vi "test-twist2d.vi"() -> (3 "All PASSED":bool)   [LabVIEW 2019]
uses:
  <vilib>/Rock Robotics/WPI/ThirdParty/JAS_Junk/TrajLib/Rotation_CreateAngle.vi
  <vilib>/Rock Robotics/WPI/ThirdParty/JAS_Junk/TrajLib/Translation_Create.vi
  <vilib>/Rock Robotics/WPI/ThirdParty/JAS_Junk/TrajLib/Trajectory_Library.lvlib
panel:
  out "T3 - Theta - 0":dbl
  out "T3 - X - 0":dbl
  out "T3 - Y - 0":dbl
  out "T2 - Equals - False":bool
  out "T1 - Equals - True":bool
  out "T0 -- Deg -- 0":dbl
  out "T0 -- y -- 0":dbl
  out "T0 -- X -- 0":dbl
  # "Twist2D Test"
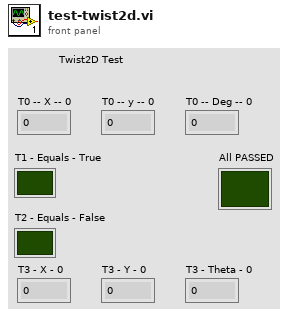
[diagram p1: front panel]
types:
  T1 = typedef "Trajectory_Library.lvlib/POSE2D.ctl" = cluster{"TRANSLATION":T2, "ROTATION":T3}
  T2 = typedef "Trajectory_Library.lvlib/TRANSLATION2D.ctl" = cluster{"X":dbl, "Y":dbl}
  T3 = typedef "Trajectory_Library.lvlib/ROTATION2D.ctl" = cluster{"VALUE":dbl, "COS":dbl, "SIN":dbl}
  T4 = typedef "Trajectory_Library.lvlib/TWIST2D.ctl" = cluster{"dX":dbl, "dY":dbl, "dTHETA":dbl}
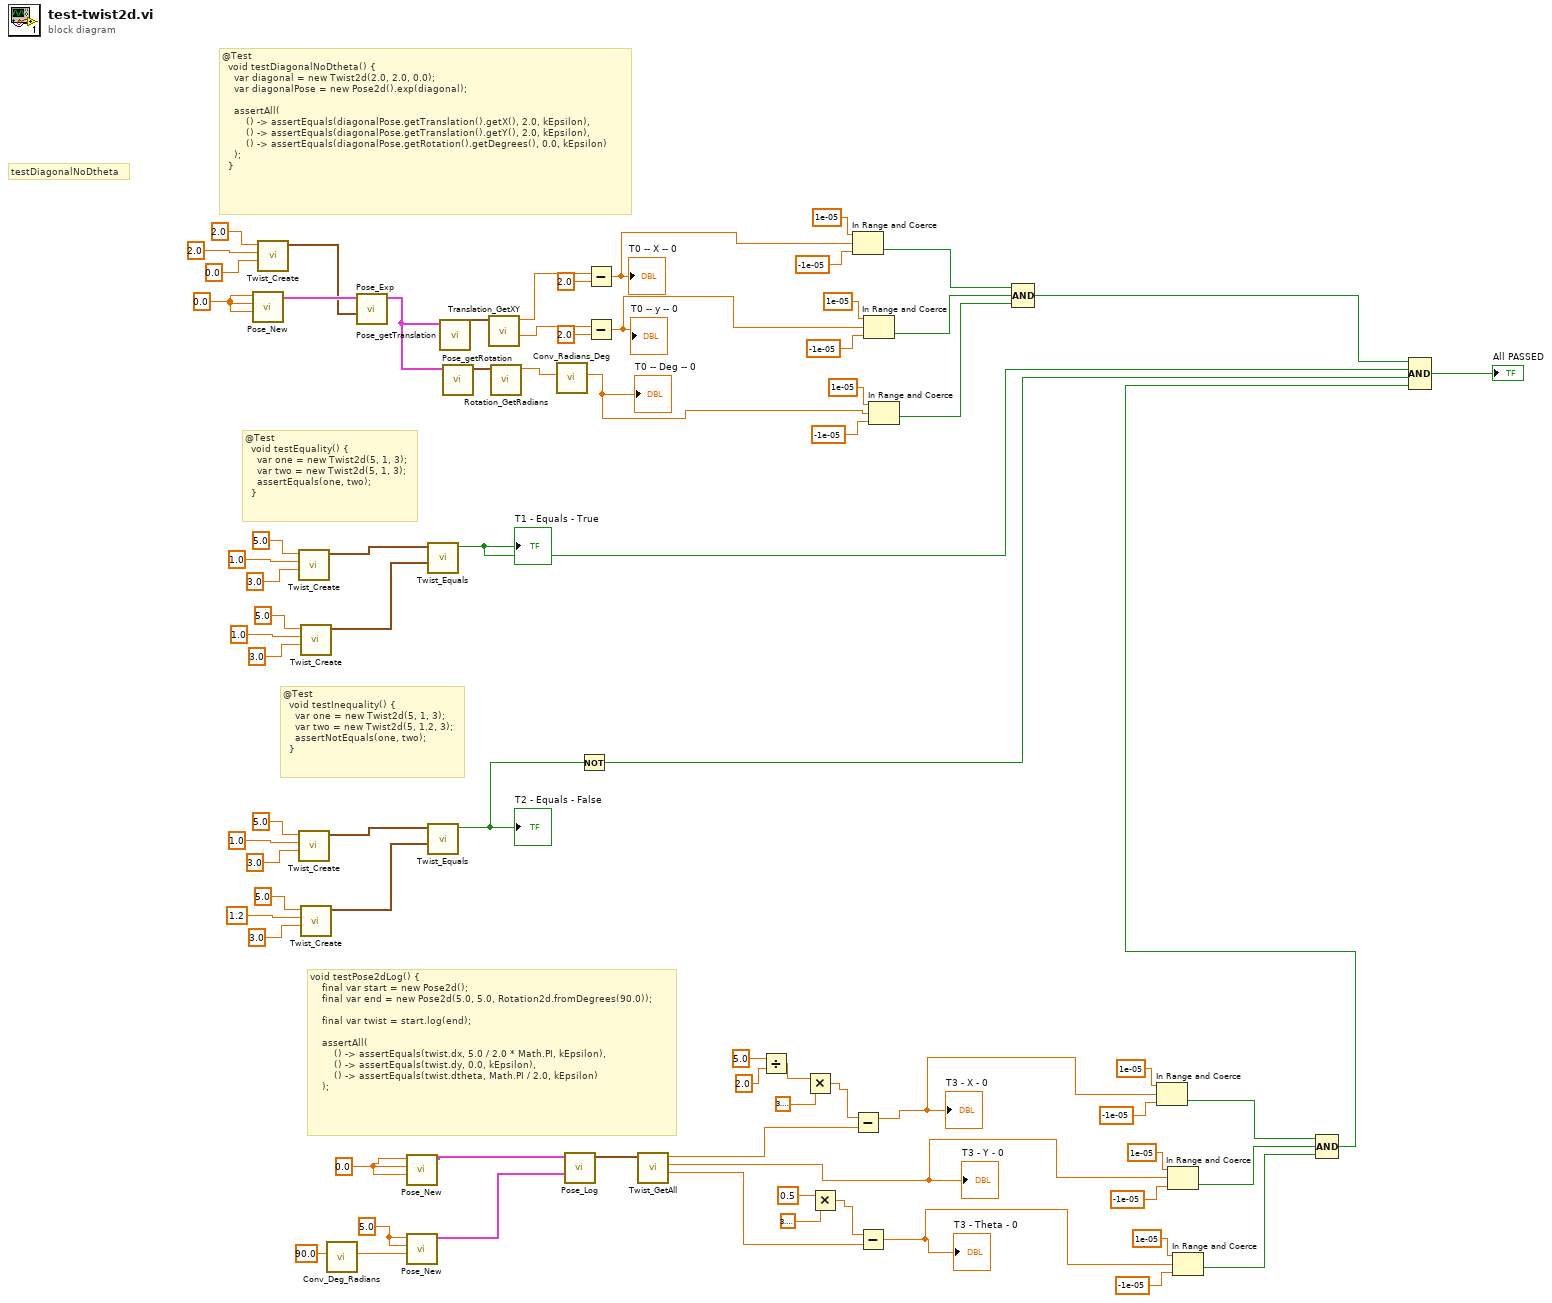
[diagram p0: block diagram]
diagram:
  w46 = 5.0 ("X")
  w31 = 0.0 ("X")
  w74 = 0.0 ("X")
  # "void testPose2dLog() {\n    final var start = new Pose2d();\n    final var end = new Pose2d(5.0, 5.0, Rotation2d.fromDegrees(90.0));\n\n    final var twist = start.log(end);\n\n    assertAll(\n        () -> assertEquals(twist.dx, 5.0 / 2.0 * Math.PI, kEpsilon),\n        () -> assertEquals(twist.dy, 0.0, kEpsilon),\n        () -> assertEquals(twist.dtheta, Math.PI / 2.0, kEpsilon)\n    );"
  # "@Test\n  void testInequality() {\n    var one = new Twist2d(5, 1, 3);\n    var two = new Twist2d(5, 1.2, 3);\n    assertNotEquals(one, two);\n  }"
  # "@Test\n  void testEquality() {\n    var one = new Twist2d(5, 1, 3);\n    var two = new Twist2d(5, 1, 3);\n    assertEquals(one, two);\n  }"
  # "@Test\n  void testDiagonalNoDtheta() {\n    var diagonal = new Twist2d(2.0, 2.0, 0.0);\n    var diagonalPose = new Pose2d().exp(diagonal);\n\n    assertAll(\n        () -> assertEquals(diagonalPose.getTranslation().getX(), 2.0, kEpsilon),\n        () -> assertEquals(diagonalPose.getTranslation().getY(), 2.0, kEpsilon),\n        () -> assertEquals(diagonalPose.getRotation().getDegrees(), 0.0, kEpsilon)\n    );\n  }"
  # "testDiagonalNoDtheta"
  n1 = call <vilib>:"Pose_New.vi"("Heading"=w74, "Y"=w74, "X"=w74) -> ("out POSe"=w73:T1)  [unwired: 8 in]
  n2 = call <vilib>:"Twist_Create.vi"("dTHETA"=0.0, "dY"=2.0, "dX"=2.0) -> ("TWIST"=w72:T4)  [unwired: 8 in]
  n3 = call <vilib>:"Twist_Create.vi"("dTHETA"=3.0, "dY"=1.0, "dX"=5.0) -> ("TWIST"=w57:T4)  [unwired: 8 in]
  n4 = call <vilib>:"Twist_Create.vi"("dTHETA"=3.0, "dY"=1.0, "dX"=5.0) -> ("TWIST"=w49:T4)  [unwired: 8 in]
  n5 = call <vilib>:"Twist_Create.vi"("dTHETA"=3.0, "dY"=1.0, "dX"=5.0) -> ("TWIST"=w56:T4)  [unwired: 8 in]
  n6 = call <vilib>:"Twist_Create.vi"("dTHETA"=3.0, "dY"=1.2, "dX"=5.0) -> ("TWIST"=w48:T4)  [unwired: 8 in]
  n7 = call <vilib>:"Conv_Deg_Radians.vi"("Degress"=90.0) -> ("Radians"=w45:dbl)  [unwired: 10 in]
  n8 = call <vilib>:"Pose_Exp.vi"("TWIST"=w72, "POSE"=w73) -> ("UpdatedPose"=w71:T1)  [unwired: 9 in]
  n9 = call <vilib>:"Pose_New.vi"("Heading"=w31, "Y"=w31, "X"=w31) -> ("out POSe"=w44:T1)  [unwired: 8 in]
  n10 = call <vilib>:"Pose_New.vi"("Heading"=w45, "Y"=w46, "X"=w46) -> ("out POSe"=w43:T1)  [unwired: 8 in]
  n11 = call <vilib>:"Twist_Equals.vi"("other TWIST"=w56, "this TWIST"=w57) -> ("Equals"=w3:bool)  [unwired: 9 in]
  "T1 - Equals - True" <- w3
  n12 = call <vilib>:"Twist_Equals.vi"("other TWIST"=w48, "this TWIST"=w49) -> ("Equals"=w4:bool)  [unwired: 9 in]
  "T2 - Equals - False" <- w4
  n13 = call <vilib>:"Pose_getTranslation.vi"("in POSE"=w71) -> ("outTRANSLATION"=w70:T2)  [unwired: 10 in]
  n14 = call <vilib>:"Pose_getRotation.vi"("in POSE"=w71) -> ("out ROTATION"=w69:T3)  [unwired: 10 in]
  n15 = call <vilib>:"Translation_GetXY.vi"("In Translation"=w70) -> ("Y"=w65:dbl, "X"=w68:dbl)  [unwired: 9 in]
  n16 = call <vilib>:"Rotation_GetRadians.vi"("in ROTATION"=w69) -> ("AngleRadians"=w64:dbl)  [unwired: 10 in]
  n17 = call <vilib>:"Conv_Radians_Deg.vi"("Radians"=w64) -> ("Degrees"=w18:dbl)  [unwired: 10 in]
  "T0 -- Deg -- 0" <- w18
  n18 = call <vilib>:"Pose_Log.vi"("end POSE"=w43, "in POSE"=w44) -> ("out TWIST"=w42:T4)  [unwired: 9 in]
  n19 = Not(x=w4) -> (.not. x?=w2:bool)
  n20 = Subtract(x=w68, y=2.0) -> (x-y=w17:dbl)
  "T0 -- X -- 0" <- w17
  n21 = Subtract(x=w65, y=2.0) -> (x-y=w19:dbl)
  "T0 -- y -- 0" <- w19
  n22 = call <vilib>:"Twist_GetAll.vi"("TWIST"=w42) -> ("dTHETA"=w32:dbl, "dY"=w6:dbl, "dX"=w36:dbl)  [unwired: 8 in]
  "T3 - Y - 0" <- w6
  n23 = Divide(x=5.0, y=2.0) -> (x/y=w38:dbl)
  n24 = Multiply(x=w38, y=3.141592653589793) -> (x*y=w37:dbl)
  n25 = Multiply(x=0.5, y=3.141592653589793) -> (x*y=w34:dbl)
  n26 = In Range and Coerce(upper limit=1e-05, x=w17, lower limit=-1e-05) -> (In Range?=w25:bool)  [unwired: 1 out]
  n27 = Subtract(x=w37, y=w36) -> (x-y=w7:dbl)
  "T3 - X - 0" <- w7
  n28 = Subtract(x=w34, y=w32) -> (x-y=w5:dbl)
  "T3 - Theta - 0" <- w5
  n29 = In Range and Coerce(upper limit=1e-05, x=w19, lower limit=-1e-05) -> (In Range?=w24:bool)  [unwired: 1 out]
  n30 = In Range and Coerce(upper limit=1e-05, x=w18, lower limit=-1e-05) -> (In Range?=w21:bool)  [unwired: 1 out]
  n31 = Compound Arithmetic op=AND(w25, w24, w21) -> (w20:bool)
  n32 = In Range and Coerce(upper limit=1e-05, x=w7, lower limit=-1e-05) -> (In Range?=w12:bool)  [unwired: 1 out]
  n33 = In Range and Coerce(upper limit=1e-05, x=w6, lower limit=-1e-05) -> (In Range?=w11:bool)  [unwired: 1 out]
  n34 = In Range and Coerce(upper limit=1e-05, x=w5, lower limit=-1e-05) -> (In Range?=w8:bool)  [unwired: 1 out]
  n35 = Compound Arithmetic op=AND(w12, w11, w8) -> (w1:bool)
  n36 = Compound Arithmetic op=AND(w20, w3, w2, w1) -> (→"All PASSED":bool)
